vi "Next JSON Value.vi"(10 "Offset":i32, 11 "JSON":string) -> (1 "<JSON>":string caption="<JSON>Value", 2 "Offset past":i32 caption="Offset past Value", 3 "Rest of Input String":string, 4 "JSON Value Type":T1)   [LabVIEW 2021, in "json.facade.lvlib"]
doc: "Gets the next JSON Value (object, array, string, number, true, false, or null)\n\n\"Offset\" should point to the start of the JSON Value, or to whitespace in front of the Value."
uses:
  json.facade.lvlib
  jsontext/JSONtext.lvlib
  jsontext/JSON Value Type.ctl
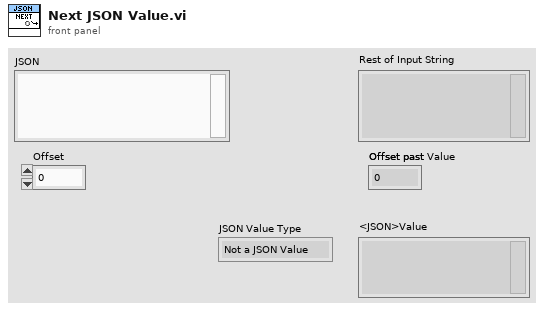
[diagram p1: front panel]
types:
  T1 = typedef "JSONtext.lvlib/JSON Value Type.ctl" = enum16{"Not a JSON Value", "JSON Object", "JSON Array", "String", "Number", "true", "false", "null"}
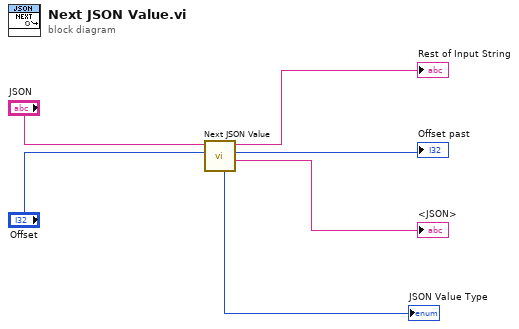
[diagram p0: block diagram]
diagram:
  n1 = call "Next JSON Value.vi"("Offset"="Offset", "JSON"="JSON") -> ("<JSON>"=→"<JSON>":string, "Offset past"=→"Offset past":i32, "Rest of Input String"=→"Rest of Input String":string, "JSON Value Type"=→"JSON Value Type":T1)  [unwired: 6 in]
